vi "Move Y Raster + B-Scan.vi"(0 "Reference In":refnum<class "_Controller.lvclass">, 1 "VISA resource name":refnum<visa-resource-name>, 2 "Source (0: Channel 1)":u16(ring) items=["Channel 1", "Channel 2", "Channel 3", "Channel 4", "Memory 1", "Memory 2", "Memory 3", "Memory 4", "Function 1", "Function 2", "Function 3", "Function 4", "Function 5", "Function 6", "Function 7", "Function 8"], 3 "Y Number of Steps":string="0", 4 "Initial Direction":bool=TRUE, 5 "Error In":errorcluster) -> (14 "Reference Out":refnum<class "_Controller.lvclass">, 16 "B-Scan":dbl[][](graph), 17 "A-Scan":waveform(dbl)[](graph), 19 "Error Out":errorcluster)   [LabVIEW 2020]
doc: "This incorporates both the motion of the machine as well as the reading from the oscilloscope in the Y direction. It then processes the incoming A-scan's mapping the values onto a B-scan. It automates the process of moving along the entire length of the Y desired length, stopping to scan at regular intervals and finally triggering the osciloscope at each scanning point and then the processing required for a B-scan.\n\nArgs:\n\nReference In: Incoming communication (reference) between LabView and the scanning rig controller\nError In: Checks for any errors with the incoming communication (reference)\nVISA Resource Name: Specifies the model of osciloscope being used \nSource (Channel): Specificies the channel that is being triggered for a reading\nY Number of Steps: Number of steps to cover the entire Y length\nInitial Direction: Direction to move in the Y direction\n\nReturns:\n\nReference Out: Output communnication (reference) between LabView and controller\nError Out: Checks for any error with output communication (reference)\nB-Scan: Resultant B-scan from all the A-scan's along that axis\nA-Scan: A-scan in the form of a waveform, note it is within a for loop so outputs multiple A-scan's in this VI alone"
uses:
  <instrlib>/Arcus Ethernet Driver 1.0.0/ArcusEthernetComm/classes/Controller/_Controller.lvclass
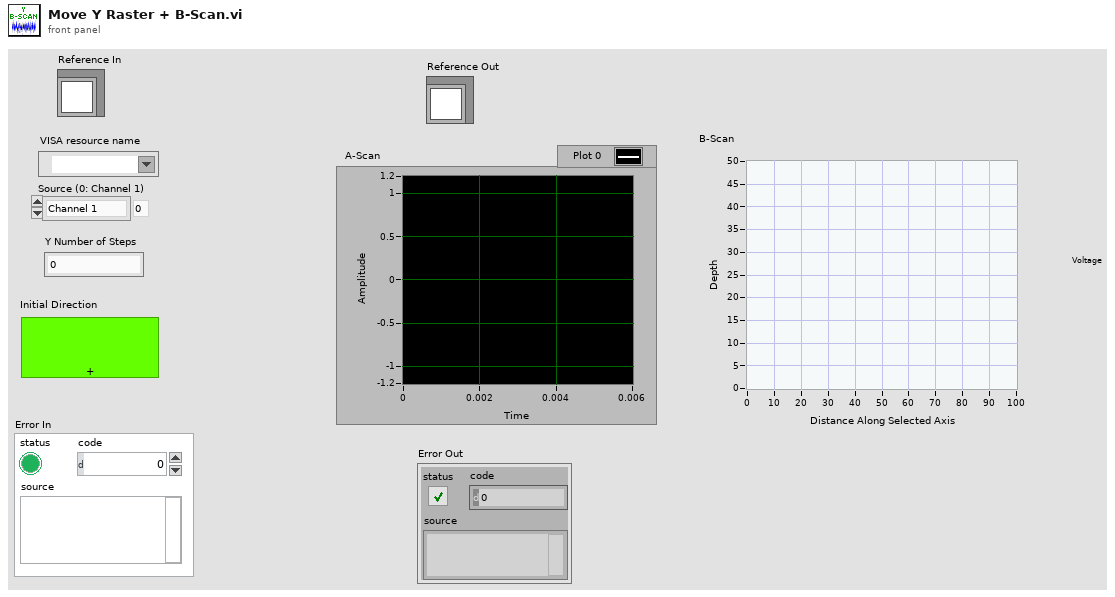
[diagram p1: front panel]
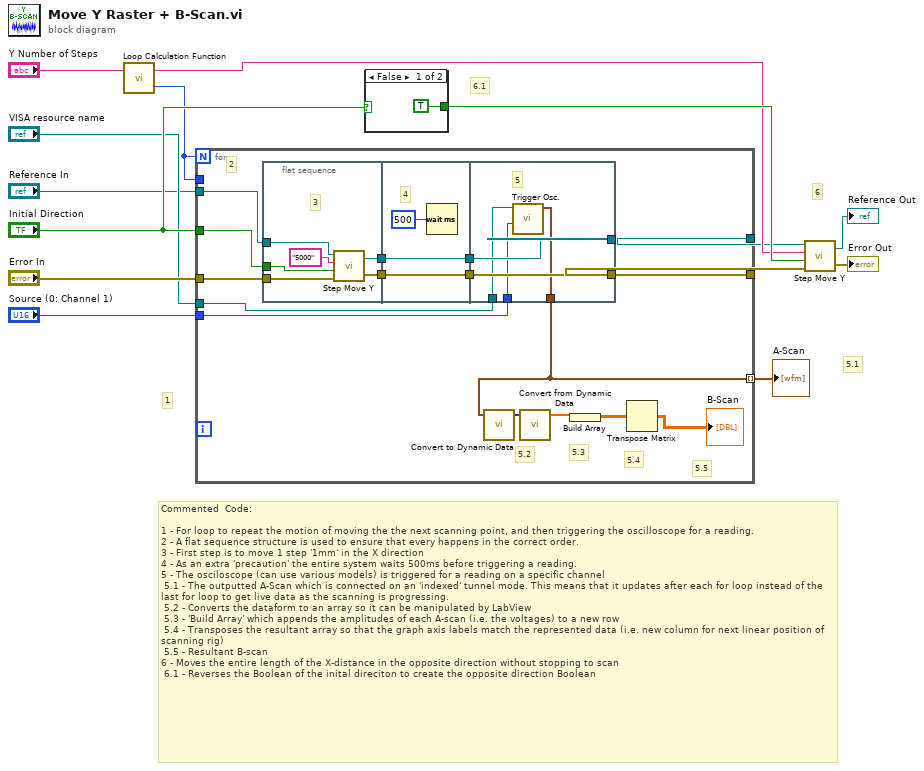
[diagram p0: block diagram]
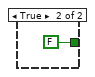
[diagram p2: hidden frame]
diagram:
  # "6.1"
  # "6"
  # "5.1"
  # "1"
  # "Commented  Code: \n\n1 - For loop to repeat the motion of moving the the next scanning point, and then triggering the oscilloscope for a reading.\n2 - A flat sequence structure is used to ensure that every happens in the correct order.\n3 - First step is to move 1 step '1mm' in the X direction\n4 - As an extra 'precaution' the entire system waits 500ms before triggering a reading.\n5 - The osciloscope (can use various models) is triggered for a reading on a specific channel\n 5.1 - The outputted A-Scan which is connected on an 'indexed' tunnel mode. This means that it updates after each for loop instead of the last for loop to get live data as the scanning is progressing. \n 5.2 - Converts the dataform to an array so it can be manipulated by LabView\n 5.3 - 'Build Array' which appends the amplitudes of each A-scan (i.e. the voltages) to a new row\n 5.4 - Transposes the resultant array so that the graph axis labels match the represented data (i.e. new column for next linear position of scanning rig)\n 5.5 - Resultant B-scan\n6 - Moves the entire length of the X-distance in the opposite direction without stopping to scan\n 6.1 - Reverses the Boolean of the inital direciton to create the opposite direction Boolean"
  n1 = call "Loop Calculation Function.vi"("Number of Steps"="Y Number of Steps") -> ("No. of Scan Points"=w1:i32)  [unwired: 1 in, 1 out]
  n2 = for {
    N: w1 -> [_]
    tunnel: [w29] -> w4
    tunnel: "Initial Direction" -> [w27]
    tunnel: [w28] -> w3
    tunnel: "Reference In" -> [w26]
    tunnel: "Error In" -> [w25]
    tunnel: "VISA resource name" -> [w24]
    tunnel: w1 -> [_]
    tunnel: "Source (0: Channel 1)" -> [w23]
    tunnel: [w21] -> w2 mode=indexing
    # "5.5"
    # "5.4"
    # "5.3"
    # "5.2"
    # "2"
    n3 = flat-sequence {
      tunnel: w27 -> [w32]
      tunnel: w26 -> [w31]
      tunnel: w25 -> [w30]
      tunnel: [w34] -> w17
      tunnel: [w33] -> w15
      tunnel: w17 -> [w38]
      tunnel: [w38] -> w16
      tunnel: w15 -> [w37]
      tunnel: [w37] -> w14
      tunnel: [w42] -> w28
      tunnel: [w43] -> w29
      tunnel: w16 -> [w43]
      tunnel: w14 -> [w42]
      tunnel: w24 -> [w41]
      tunnel: w23 -> [w40]
      tunnel: [w39] -> w21
      frame #0 {
        # "3"
        n4 = call "Step Move Y.vi"("Error In"=w30, "Direction"=w32, "No. of Y Steps"="5000" ("X Steps"), "Reference In"=w31) -> ("Error Out"=w33:errorcluster, "Reference Out"=w34:refnum<class "_Controller.lvclass">)
      }
      frame #1 {
        # "4"
        n5 = Wait (ms)(milliseconds to wait=u32 500) -> ()  [unwired: 1 out]
      }
      frame #2 {
        # "5"
        n6 = call "Trigger Osc..vi"("Source (0: Channel 1)"=w40, "VISA resource name"=w41) -> ("Waveform Data"=w39:waveform(dbl))  [unwired: 9 in]
      }
    }
    n7 = call "Convert to Dynamic Data"("Waveform"=w21) -> ("Dynamic Data Type"=w22:dynamicdata)  [unwired: 3 in]
    n8 = call "Convert from Dynamic Data"("Dynamic Data Type"=w22) -> ("Array"=w20:dbl[])  [unwired: 3 in]
    n9 = Build Array(w20) -> (w19:dbl[][])
    n10 = Transpose Matrix(1:w19) -> (0:→"B-Scan":dbl[][])
  }
  "A-Scan" <- w2
  n11 = case shown="False" "Initial Direction" {
    tunnel: [TRUE FALSE] -> w12
    frame False {
    }
    frame True {
    }
  }
  n12 = call "Step Move Y.vi"("Error In"=w3, "Direction"=w12, "No. of Y Steps"="Y Number of Steps", "Reference In"=w4) -> ("Error Out"=→"Error Out":errorcluster, "Reference Out"=→"Reference Out":refnum<class "_Controller.lvclass">)
